vi "Get Value by Array (String Value).vi"(8 "error in (no error)":errorcluster, 10 "Keys":string[](array[string]), 11 "JSON Object in":refnum<class "JSON Object.lvclass">) -> (0 "error out":errorcluster, 2 "value":string)   [LabVIEW 2015, in "LVJSON.lvlib" / "JSON Object.lvclass"]
uses:
  JSON Object.lvclass
  Get Value by Array (String).vi
  JSON String/Read value (String).vi
  JSON Basic Type/JSON Basic Type.lvclass
  JSON String/JSON String.lvclass
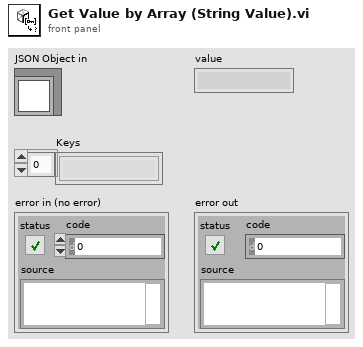
[diagram p1: front panel]
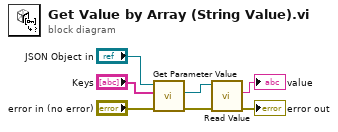
[diagram p0: block diagram]
diagram:
  n1 = call-poly "Get Parameter Value.vi"("error in (no error)"="error in (no error)", "Keys"="Keys", "JSON Object in"="JSON Object in") -> ("error out"=w1:errorcluster, "JSON String out"=w2:refnum<class "JSON String.lvclass">)  [unwired: 7 in]
  n2 = call-poly "Read Value.vi"("error in (no error)"=w1, "JSON String in"=w2) -> ("error out"=→"error out":errorcluster, "value"=→"value":string)  [unwired: 8 in]
